vi "Close connection.vi"(0 "System no.":i32=1 min=1 step=1, 2 "Close DaisyChain":bool, 5 "error in":errorcluster) -> (14 "Was connected?":bool, 19 "error out":errorcluster)   [LabVIEW 2014]
doc: "This VI checks if the connection to the selected system is already open and, if it is, it closes this connection. \n\nValid for all systems."
uses:
  GCS_LabVIEW/Low Level/Communication.llb/Available interfaces.ctl
  GCS_LabVIEW/Low Level/Communication.llb/Available DLLs.ctl
  GCS_LabVIEW/Low Level/Communication.llb/Global1.vi
  GCS_LabVIEW/Low Level/Communication.llb/Global DaisyChain.vi
panel:
  out "DLL for Device":T1 items=["C-843", "C-844", "E-710", "C-843.PM", "C-865", "E-761", "Mercury", "E-755", "E-753", "C-866", "E-712", "E-725", "E-861", "C-867", "E-517", "E-816", "E-709", "PI_GCS2_DLL", "HydraPollux"]
  out "Interface":T2 items=["RS232", "GPIB", "DLL", "TCP-IP", "USB", "Analog"]
  out "VISA resource name":refnum<visa-resource-name>
  # "This vi checks if the connection to the selected system\nis already open and, if it is, it closes this connection."
  # "Communication setup indicators (for troubleshooting):"
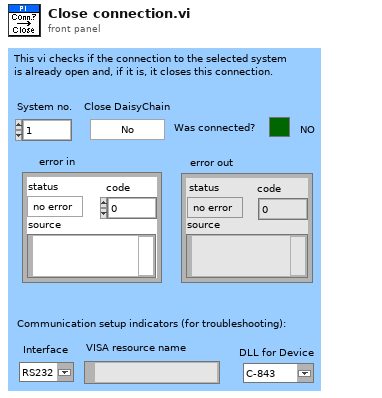
[diagram p1: front panel]
types:
  T1 = typedef "Available DLLs.ctl" = u16
  T2 = typedef "Available interfaces.ctl" = u16
  T3 = cluster{"RS232 Portnumber":i32, "Timeout":i32, "RS232 Baud rate":u32, "Interface":T2, "GPIB Bus":i32, "GPIB Address":i32, "GPIB Mode":i32}[]
  T4 = typedef "Available DLL interfaces.ctl" = u16
  T5 = cluster{"DLL for Device":T1, "DLL Interface":T4, "Parameter":string}[]
  T6 = cluster{"RS232 Portnumber":i32, "Timeout":i32, "RS232 Baud rate":u32, "Interface":T2, "GPIB Bus":i32, "GPIB Address":i32, "GPIB Mode":i32}
  T7 = cluster{"DLL for Device":T1, "DLL Interface":T4, "Parameter":string}
  T8 = enum16{"C844_IsDLLAvailable", "C844_ConnectRS232", "C844_ConnectNIgpib", "C844_IsConnected", "C844_CloseConnection", "C844_GcsCommandset", "C844_GetError", "C844_GcsGetAnswerSize", "C844_GcsGetAnswer", "C843_IsDLLAvailable", "C843_Connect", "C843_IsConnected", "C843_CloseConnection", "C843_GcsCommandset", "C843_GetError", "C843_GcsGetAnswerSize", "C843_GcsGetAnswer", "E710_IsDLLAvailable", "E710_ConnectRS232", "E710_ConnectNIgpib", "E710_IsConnected", "E710_CloseConnection", "E710_GcsCommandset", "E710_GetError", "E710_GcsGetAnswerSize", "E710_GcsGetAnswer", "C843_PM_IsDLLAvailable", "C843_PM_Connect", "C843_PM_IsConnected", "C843_PM_CloseConnection", "C843_PM_GcsCommandset", "C843_PM_GetError", "C843_PM_GcsGetAnswerSize", "C843_PM_GcsGetAnswer", "C843_PM_GetCurrentBoardID", "C843_GetCurrentBoardID", "C865_IsDLLAvailable", "C865_ConnectRS232", "C865_IsConnected", "C865_CloseConnection", "C865_GcsCommandset", "C865_GetError", "C865_GcsGetAnswerSize", "C865_GcsGetAnswer", "C865_GetCurrentInterfaceID", "E761_ConnectPciBoard", "DefineSystem", "CloseConnection", "IsConnected", "ConnectRS232", "ConnectNIgpib", "ConnectPciBoard", "ConnectTCPIP", "GetError", "GcsCommandset", "GCSGetAnswerSize", "GcsGetAnswer"}
  T9 = enum16{"C844_IsDLLAvailable", "C844_ConnectRS232", "C844_ConnectNIgpib", "C844_IsConnected", "C844_CloseConnection", "C844_GcsCommandset", "C844_GetError", "C844_GcsGetAnswerSize", "C844_GcsGetAnswer", "C843_IsDLLAvailable", "C843_Connect", "C843_IsConnected", "C843_CloseConnection", "C843_GcsCommandset", "C843_GetError", "C843_GcsGetAnswerSize", "C843_GcsGetAnswer", "E710_IsDLLAvailable", "E710_ConnectRS232", "E710_ConnectNIgpib", "E710_IsConnected", "E710_CloseConnection", "E710_GcsCommandset", "E710_GetError", "E710_GcsGetAnswerSize", "E710_GcsGetAnswer", "C843_PM_IsDLLAvailable", "C843_PM_Connect", "C843_PM_IsConnected", "C843_PM_CloseConnection", "C843_PM_GcsCommandset", "C843_PM_GetError", "C843_PM_GcsGetAnswerSize", "C843_PM_GcsGetAnswer", "C843_PM_GetCurrentBoardID", "C843_GetCurrentBoardID", "C865_IsDLLAvailable", "C865_ConnectRS232", "C865_IsConnected", "C865_CloseConnection", "C865_GcsCommandset", "C865_GetError", "C865_GcsGetAnswerSize", "C865_GcsGetAnswer", "C865_GetCurrentInterfaceID", "E761_ConnectPciBoard", "DefineSystem", "CloseConnection", "IsConnected", "ConnectRS232", "ConnectNIgpib", "ConnectPciBoard", "ConnectTCPIP", "GetError", "GcsCommandset", "GCSGetAnswerSize", "GcsGetAnswer", "CloseDaisyChain", "OpenRS232DaisyChain", "ConnectDaisyChainDevice"}
  T10 = cluster{"No. of devices":i32, "Port ID":i32, "Devices":string[], "Description":string}[]
  T11 = cluster{"No. of devices":i32, "Port ID":i32, "Devices":string[], "Description":string}
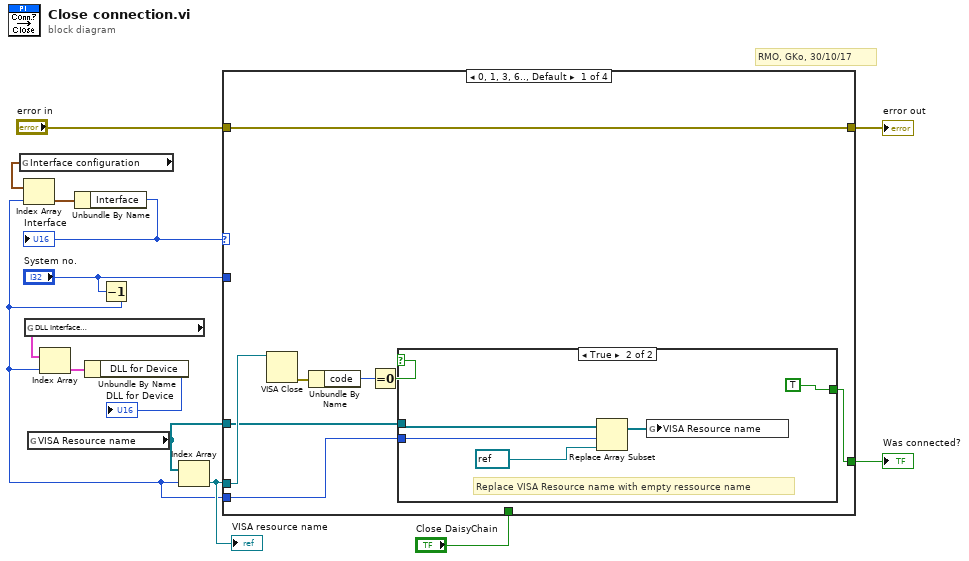
[diagram p0: block diagram]
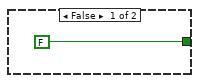
[diagram p2: hidden frame]
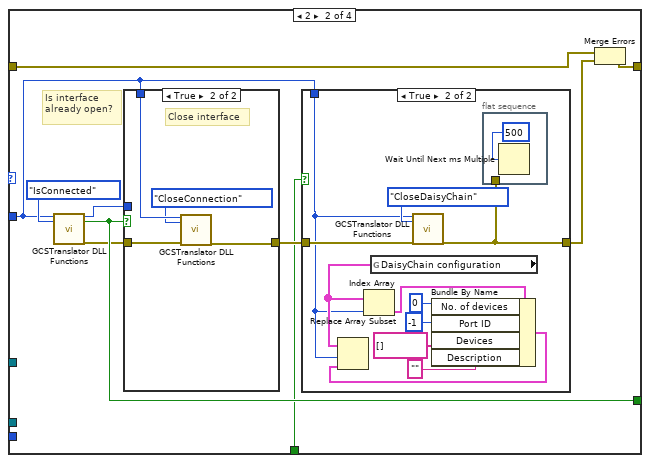
[diagram p3: hidden frame]
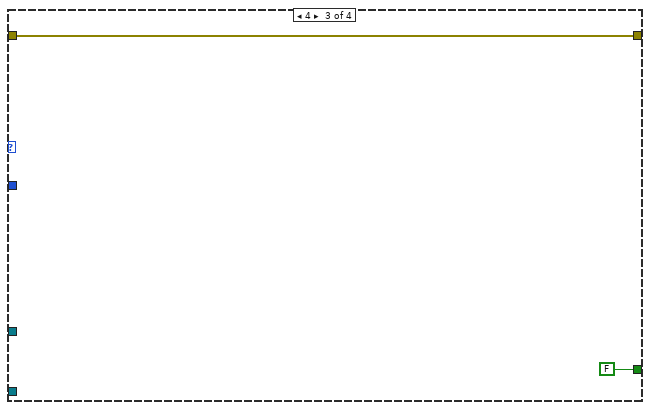
[diagram p6: hidden frame]
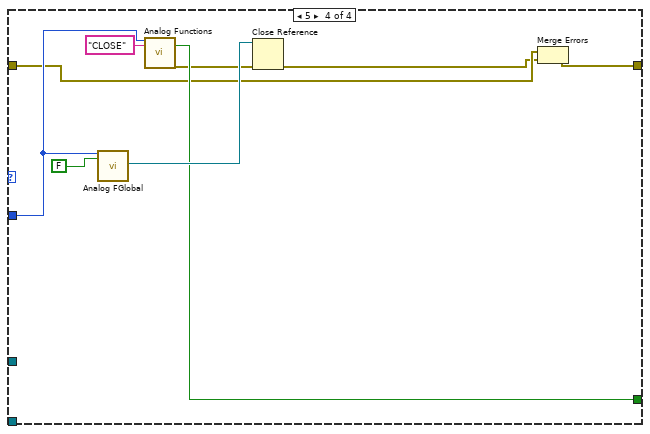
[diagram p7: hidden frame]
diagram:
  # "RMO, GKo, 30/10/17"
  n1 = global read "Global1.vi" "Interface configuration"() -> (w11:T3)
  n2 = global read "Global1.vi" "DLL Interface\nConfiguration"() -> (w4:T5)
  n3 = global read "Global1.vi" "VISA Resource name"() -> (w2:refnum<visa-resource-name>[])
  n4 = Decrement(x="System no.") -> (x-1=w1:i32)
  n5 = Index Array(array=w11, index=w1) -> (element=w10:T6)
  n6 = Index Array(array=w4, index=w1) -> (element=w5:T7)
  n7 = Unbundle By Name(w10) -> ("Interface"=w7:T2)
  "Interface" <- w7
  n8 = Unbundle By Name(w5) -> ("DLL for Device"=→"DLL for Device":T1)
  n9 = Index Array(array=w2, index=w1) -> (element=w8:refnum<visa-resource-name>)
  "VISA resource name" <- w8
  n10 = case shown="0, 1, 3, 6.., Default" w7 {
    tunnel: "error in" -> [w21 w30 w58 w60]
    tunnel: [w21 w31 w58 w61] -> w13
    tunnel: "System no." -> [_ w32 _ w65]
    tunnel: [w20 w38 FALSE ("Boolean output") w63] -> w12
    tunnel: w8 -> [w22 _ _ _]
    tunnel: "Close DaisyChain" -> [_ w33 _ _]
    tunnel: w2 -> [w16 _ _ _]
    tunnel: w1 -> [w15 _ _ _]
    frame 0, 1, 3, 6.., Default {
      n11 = VISA Close(VISA resource name=w22) -> (error out=w19:errorcluster)  [unwired: 1 in]
      n12 = Unbundle By Name(w19) -> ("code"=w18:i32)
      n13 = Equal To 0?(x=w18) -> (x = 0?=w17:bool)
      n14 = case shown="True" w17 {
        tunnel: [FALSE ("Boolean output") TRUE ("Boolean output")] -> w20
        tunnel: w16 -> [_ w27]
        tunnel: w15 -> [_ w26]
        frame False {
        }
        frame True {
          # "Replace VISA Resource name with empty ressource name"
          n15 = Replace Array Subset(array=w27, new element=refnum<visa-resource-name> refnum ("new element/subarray"), index=w26) -> (w24:refnum<visa-resource-name>[])
          n16 = global write "Global1.vi" "VISA Resource name"(w24) -> ()
        }
      }
    }
    frame 2 {
      # "Is interface\nalready open?"
      n17 = call "GCSTranslator DLL Functions.vi"("System no."=w32, "Function"=T8."IsConnected") -> ("DLL I32 Return value"=w36:i32, "Boolean output"=w38:bool, "error out"=w37:errorcluster)  [unwired: 5 in, 10 out]
      n18 = case shown="True" w38 {
        tunnel: w37 -> [w52 w56]
        tunnel: [w52 w55] -> w34
        tunnel: w32 -> [_ w54]
        tunnel: w36 -> [_ _]
        frame False {
        }
        frame True {
          # "Close interface"
          n19 = call "GCSTranslator DLL Functions.vi"("System no."=w54, "Function"=T8."CloseConnection", "error in"=w56) -> ("error out"=w55:errorcluster)  [unwired: 4 in, 12 out]
        }
      }
      n20 = case shown="True" w33 {
        tunnel: w34 -> [w39 w49]
        tunnel: [w39 w48] -> w29
        tunnel: w32 -> [_ w40]
        frame False {
        }
        frame True {
          n21 = global read "Global DaisyChain.vi" "DaisyChain configuration"() -> (w46:T10)
          n22 = Index Array(array=w46, index=w40) -> (element=w41:T11)
          n23 = call "GCSTranslator DLL Functions.vi"("System no."=w40, "Function"=T9."CloseDaisyChain", "error in"=w49) -> ("error out"=w48:errorcluster)  [unwired: 4 in, 12 out]
          n24 = Bundle By Name(cluster=w41, "No. of devices"=0, "Port ID"=-1, "Devices"=string[] [], "Description"="") -> (w47:T11)
          n25 = Replace Array Subset(array=w46, new element=w47, index=w40) -> ()  [unwired: 1 out]
          n26 = flat-sequence {
            tunnel: w48 -> [_]
            frame #0 {
              n27 = Wait Until Next ms Multiple(millisecond multiple=u32 500) -> ()  [unwired: 1 out]
            }
          }
        }
      }
      n28 = Merge Errors(w30, w29) -> (w31:errorcluster)
    }
    frame 4 {
    }
    frame 5 {
      n29 = call "Analog FGlobal.vi"("System no."=w65, "Read(F)/Write"=FALSE) -> ("VI ref out"=w66:refnum<vi>)  [unwired: 1 in, 16 out]
      n30 = call "Analog Functions.vi"("System no."=w65, "String to send"="CLOSE") -> ("Boolean output"=w63:bool, "error out"=w62:errorcluster)  [unwired: 5 in, 11 out]
      n31 = Close Reference(reference=w66, error in (no error)=w62) -> (error out=w59:errorcluster)
      n32 = Merge Errors(w60, w59) -> (w61:errorcluster)
    }
  }
  "error out" <- w13
  "Was connected?" <- w12
